vi "tele_treshold.vi"(6 "lower limit":dbl=40.0, 7 "upper limit":dbl=100.0, 9 "Right in":i8, 11 "Left in":i8) -> (2 "Right out":i8, 3 "Left out":i8)   [LabVIEW 2012, in "BlockParty4150.lvrbt"]
uses:
  BlockParty4150/BlockParty4150.lvrbt
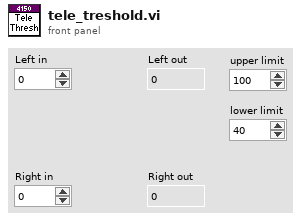
[diagram p1: front panel]
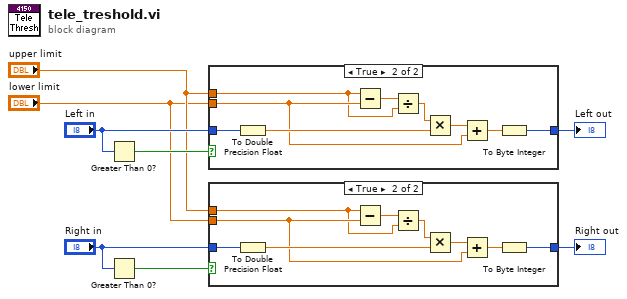
[diagram p0: block diagram]
diagram:
  n1 = Greater Than 0?(x="Left in") -> (x > 0?=w6:bool)
  n2 = Greater Than 0?(x="Right in") -> (x > 0?=w5:bool)
  n3 = case shown="True" w6 {
    tunnel: [w9 w14] -> w8
    tunnel: "Left in" -> [w9 w12]
    tunnel: "lower limit" -> [_ w11]
    tunnel: "upper limit" -> [_ w10]
    frame False {
    }
    frame True {
      n4 = To Double Precision Float(number=w12) -> (double precision float=w13:dbl)
      n5 = Subtract(x=w10, y=w11) -> (x-y=w18:dbl)
      n6 = Divide(x=w18, y=w10) -> (x/y=w17:dbl)
      n7 = Multiply(x=w17, y=w13) -> (x*y=w16:dbl)
      n8 = Add(x=w16, y=w11) -> (x+y=w15:dbl)
      n9 = To Byte Integer(number=w15) -> (8bit integer=w14:i8)
    }
  }
  "Left out" <- w8
  n10 = case shown="True" w5 {
    tunnel: [w19 w24] -> w3
    tunnel: "Right in" -> [w19 w22]
    tunnel: "lower limit" -> [_ w21]
    tunnel: "upper limit" -> [_ w20]
    frame False {
    }
    frame True {
      n11 = To Double Precision Float(number=w22) -> (double precision float=w23:dbl)
      n12 = Subtract(x=w20, y=w21) -> (x-y=w28:dbl)
      n13 = Divide(x=w28, y=w20) -> (x/y=w27:dbl)
      n14 = Multiply(x=w27, y=w23) -> (x*y=w26:dbl)
      n15 = Add(x=w26, y=w21) -> (x+y=w25:dbl)
      n16 = To Byte Integer(number=w25) -> (8bit integer=w24:i8)
    }
  }
  "Right out" <- w3
